vi "Wait For Theta.vi"(4 "error in (no error)":errorcluster, 5 "Theta Setpoint":dbl, 6 "Delay (s)":u32=5, 7 "Instrument Ref In":refnum<k24>) -> (0 "error out":errorcluster, 2 "Current Theta":dbl, 3 "Instrument Ref Out":refnum<k24>)   [LabVIEW 2020]
uses:
  C:/Users/qmgmit/Desktop/Shivam/dev/QDInstrument/QDInstrument.dll
  dev/QDInstrument/QDInstrument.dll
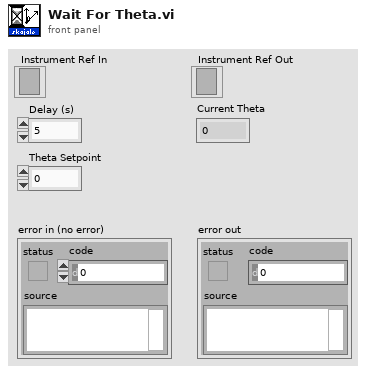
[diagram p1: front panel]
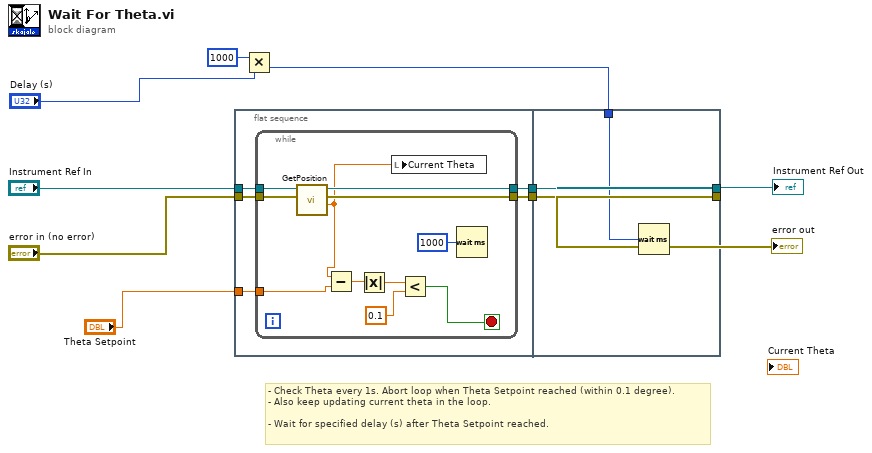
[diagram p0: block diagram]
diagram:
  # "- Check Theta every 1s. Abort loop when Theta Setpoint reached (within 0.1 degree).\n- Also keep updating current theta in the loop.\n\n- Wait for specified delay (s) after Theta Setpoint reached."
  n1 = flat-sequence {
    tunnel: "Instrument Ref In" -> [w15]
    tunnel: "error in (no error)" -> [w13]
    tunnel: [w14] -> w6
    tunnel: [w12] -> w5
    tunnel: "Theta Setpoint" -> [w11]
    tunnel: [w28] -> w7
    tunnel: [w29] -> w9
    tunnel: w6 -> [w29]
    tunnel: w5 -> [w28]
    tunnel: w3 -> [w27]
    frame #0 {
      n2 = while {
        tunnel: w15 -> [w26]
        tunnel: [w25] -> w14
        tunnel: w13 -> [w24]
        tunnel: [w23] -> w12
        tunnel: w11 -> [w20]
        stop <- w17 stop-if-true
        n3 = call "GetPosition.vi"("error in (no error)"=w24, "Instrument Ref In"=w26) -> ("Position"=w21:dbl, "error out"=w23:errorcluster, "Instrument Ref Out"=w25:refnum<k24>)  [unwired: 2 in, 1 out]
        n4 = Subtract(x=w21, y=w20) -> (x-y=w19:dbl)
        n5 = Absolute Value(x=w19) -> (abs(x)=w18:dbl)
        n6 = local write "Current Theta"(w21) -> ()
        n7 = Less?(x=w18, y=0.1) -> (x < y?=w17:bool)
        n8 = Wait (ms)(milliseconds to wait=u32 1000) -> ()  [unwired: 1 out]
      }
    }
    frame #1 {
      n9 = Wait (ms)(milliseconds to wait=w27) -> ()  [unwired: 1 out]
    }
  }
  n10 = Multiply(x=u32 1000, y="Delay (s)") -> (x*y=w3:u32)
  "Instrument Ref Out" <- w9
  "error out" <- w7
